vi "Error Query.vi"(8 "error in":errorcluster, 11 "VISA resource name":refnum<visa-resource-name>) -> (0 "error out":errorcluster, 1 "Error Message":string, 2 "Error Code":i32[](array[numeric]), 3 "VISA resource name out":refnum<visa-resource-name>)   [LabVIEW 2020, in "IT-M3400.lvlib"]
doc: "Queries the instrument for any errors in the instrument's error queue. It will continue to read errors until all errors have been read from the instrument. Any errors will be returned in the <B>error out</B> control.\n\n<B>Note:</B>\nThis VI is called automatically by most driver VIs so it is not usually necessary to call this in an application."
uses:
  <instrlib>/IT-M3400/IT-M3400.lvlib
panel:
  # "EDIT: Note: The Error Query VI is included as a subVI in all driver VIs except low-level API VIs. If the instrument does not support error query, then remove the VI and remove subVI calls in each instrument driver VI that calls it."
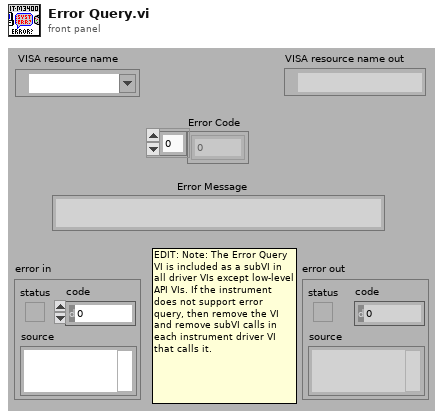
[diagram p1: front panel]
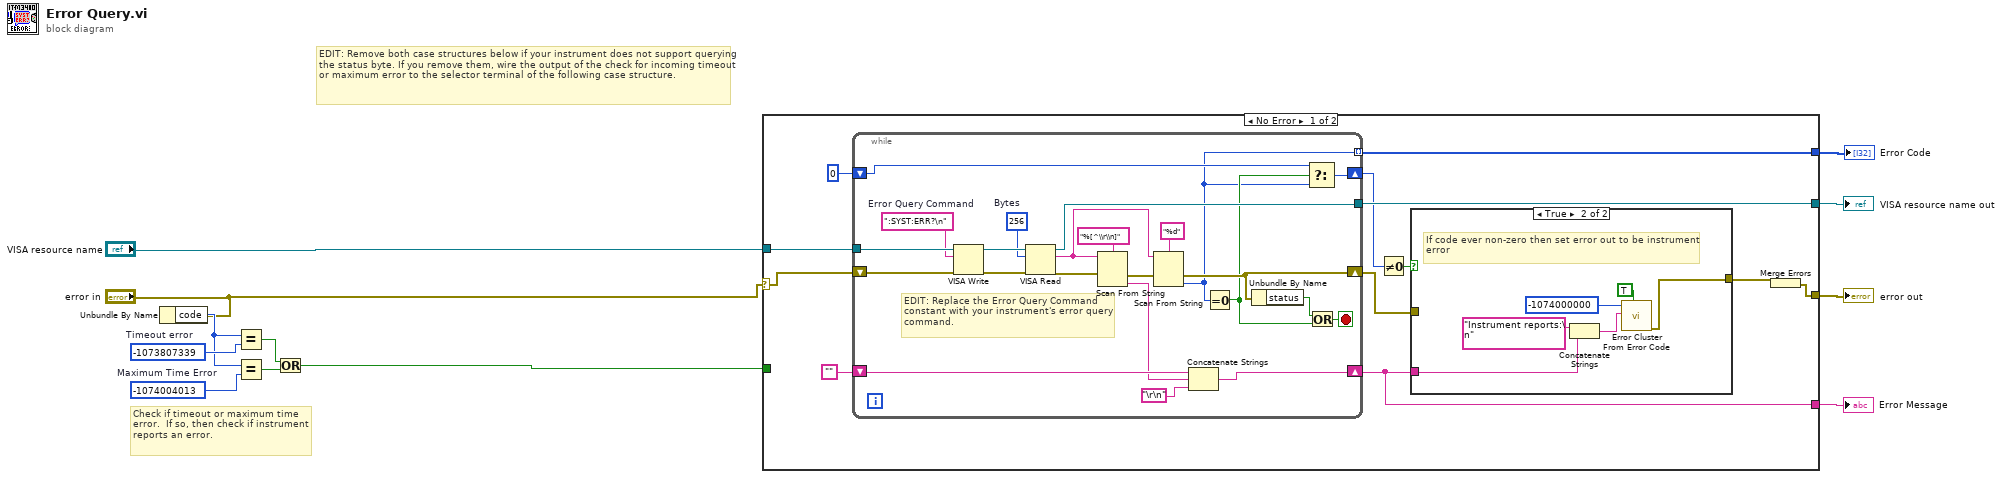
[diagram p0: block diagram]
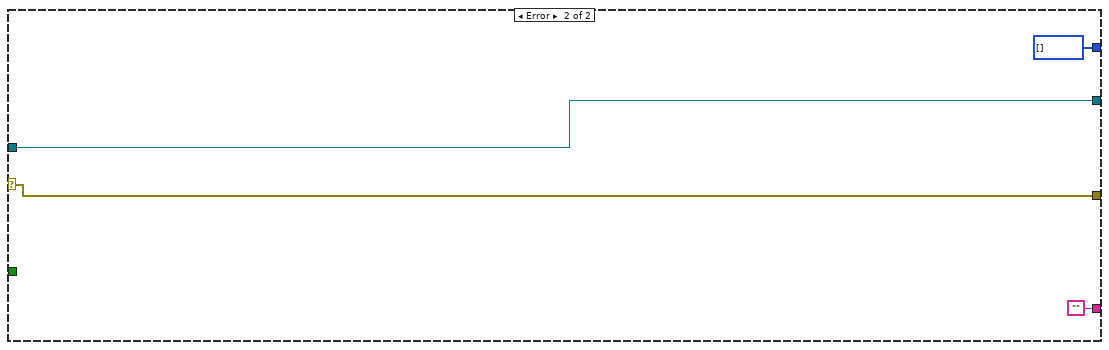
[diagram p3: hidden frame]
diagram:
  w6 = -1074004013  # Maximum Time Error
  w8 = -1073807339  # Timeout error
  # "Check if timeout or maximum time error.  If so, then check if instrument reports an error."
  # "EDIT: Remove both case structures below if your instrument does not support querying the status byte. If you remove them, wire the output of the check for incoming timeout or maximum error to the selector terminal of the following case structure."
  n1 = Unbundle By Name("error in") -> ("code"=w7:i32)
  n2 = Equal?(x=w7, y=w8) -> (x = y?=w4:bool)
  n3 = Equal?(x=w7, y=w6) -> (x = y?=w5:bool)
  n4 = Or(x=w4, y=w5) -> (x .or. y?=w1:bool)
  n5 = case shown="No Error" "error in" {
    selector: "error in" -> [w13 w55]
    tunnel: [w24 w58] -> w12
    tunnel: "VISA resource name" -> [w23 w58]
    tunnel: [w21 w55] -> w11
    tunnel: [w16 ""] -> w10
    tunnel: [w15 i32[] []] -> w9
    tunnel: w1 -> [_ _]
    frame No Error {
      n6 = while {
        tunnel: [w54] -> w24
        tunnel: w23 -> [w53]
        shift-right: [w41] -> w16
        shift-left: "" -> [w44]
        shift-right: [w39] -> w17
        shift-left: 0 -> [w40]
        shift-right: [w37] -> w14
        shift-left: w13 -> [w38]
        tunnel: [w32] -> w15 mode=indexing
        stop <- w47 stop-if-true
        w51 = u32 256  # Bytes
        w49 = ":SYST:ERR?\n"  # Error Query Command
        # "EDIT: Replace the Error Query Command constant with your instrument's error query command."
        n7 = VISA Write(VISA resource name=w53, write buffer=w49, error in (no error)=w38) -> (VISA resource name out=w52:refnum<visa-resource-name>, error out=w50:errorcluster)  [unwired: 1 out]
        n8 = VISA Read(VISA resource name=w52, byte count=w51, error in (no error)=w50) -> (VISA resource name out=w54:refnum<visa-resource-name>, read buffer=w45:string, error out=w36:errorcluster)  [unwired: 1 out]
        n9 = Scan From String(format string="%[^\\r\\n]", input string=w45, error in=w36) -> (error out=w35:errorcluster, output 1=w42:string)  [unwired: 2 in, 2 out]
        n10 = Scan From String(format string="%d", input string=w45, error in=w35) -> (error out=w37:errorcluster, output 1=w32:i32)  [unwired: 2 in, 2 out]
        n11 = Concatenate Strings(w44, w42, "\r\n") -> (w41:string)
        n12 = Equal To 0?(x=w32) -> (x = 0?=w33:bool)
        n13 = Unbundle By Name(w37) -> ("status"=w34:bool)
        n14 = Select(t=w40, s=w33, f=w32) -> (s? t:f=w39:i32)
        n15 = Or(x=w34, y=w33) -> (x .or. y?=w47:bool)
      }
      n16 = Not Equal To 0?(x=w17) -> (x != 0?=w19:bool)
      n17 = case shown="True" w19 {
        tunnel: w16 -> [_ w30]
        tunnel: [w25 w26] -> w18
        tunnel: w14 -> [w25 _]
        frame False {
        }
        frame True {
          # "If code ever non-zero then set error out to be instrument error"
          n18 = Concatenate Strings("Instrument reports:\n" ("Source"), w30) -> (w27:string)
          n19 = call <vilib>:"Error Cluster From Error Code.vi"("show call chain? (False)"=TRUE, "error message (\"\")"=w27, "error code (0)"=-1074000000 ("Code")) -> ("error out"=w26:errorcluster)  [unwired: 6 in]
        }
      }
      n20 = Merge Errors(w18) -> (w21:errorcluster)
    }
    frame Error {
    }
  }
  "VISA resource name out" <- w12
  "error out" <- w11
  "Error Message" <- w10
  "Error Code" <- w9
